vi "Configure Module.vi"(8 "error in (no error)":errorcluster, 10 "IOV ref in":refnum<k21>, 11 "Module Template in":refnum<class "9401.lvclass">) -> (0 "error out":errorcluster, 2 "IOV ref out":refnum<k21>, 3 "Module Template out":refnum<class "9401.lvclass">)   [LabVIEW 2017, in "Modules.lvlib" / "9401.lvclass"]
uses:
  9401.lvclass
  C:/Users/rzoeller/Documents/ni-official/niveristand-scan-engine-module-libraries/Source/SD Module/SD Module.lvclass
  9401.lvclass/9401.ctl
  SD Module/SD Module.lvclass
  <resource>/objmgr/cRIO.rc
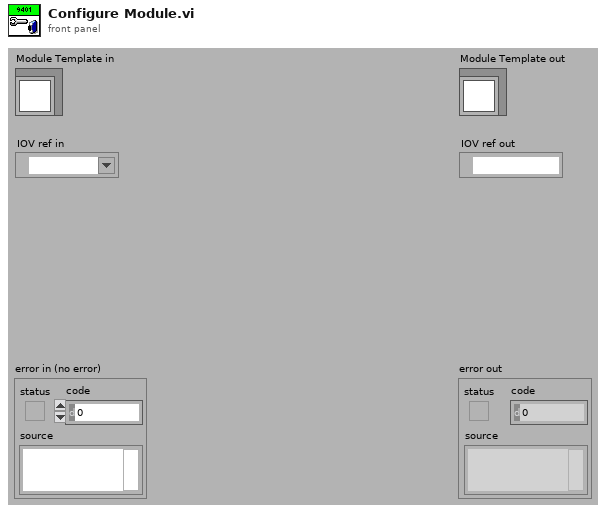
[diagram p1: front panel]
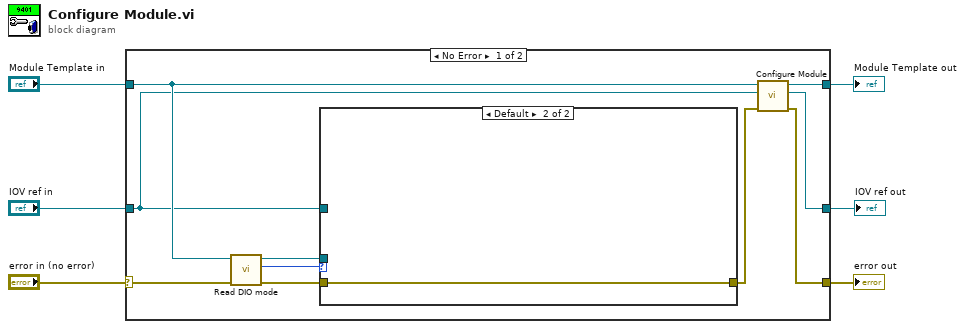
[diagram p0: block diagram]
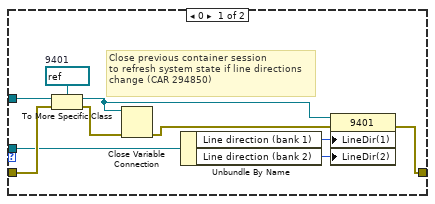
[diagram p2: hidden frame]
diagram:
  n1 = case shown="No Error" "error in (no error)" {
    selector: "error in (no error)" -> [w15 w30]
    tunnel: [w11 w30] -> w5
    tunnel: [w7 w29] -> w3
    tunnel: "Module Template in" -> [w10 w29]
    tunnel: "IOV ref in" -> [w9 w28]
    tunnel: [w8 w28] -> w1
    frame No Error {
      n2 = call "Read DIO mode.vi"("error in (no error)"=w15, "SD Module in"=w10) -> ("error out"=w13:errorcluster, "DIO mode"=w14:u32, "SD Module out"=w16:refnum<class "9401.lvclass">)  [unwired: 7 in]
      n3 = case shown="Default" w14 {
        tunnel: [w17 w27] -> w12
        tunnel: w9 -> [w25 _]
        tunnel: w16 -> [w18 _]
        tunnel: w13 -> [w19 w27]
        frame 0 {
          w26 = refnum<k21> refnum  # 9401
          # "Close previous container session\nto refresh system state if line directions\nchange (CAR 294850)"
          n4 = To More Specific Class(target class=w26, reference=w25, error in=w19) -> (specific class reference=w20:refnum<k21>, error out=w22:errorcluster)
          n5 = Close Variable Connection(8:w22, 11:w20) -> (0:w21:errorcluster)
          n6 = Unbundle By Name(w18) -> ("Line direction (bank 1)"=w24:u32, "Line direction (bank 2)"=w23:u32)
          n7 = property class="9401"(reference=w20, error in=w21, "LineDir(1)"=w24, "LineDir(2)"=w23) -> (error out=w17:errorcluster)  [unwired: 1 out]
        }
        frame Default {
        }
      }
      n8 = call-parent "Configure Module.vi"("error in (no error)"=w12, "IOV ref in"=w9, "Module Template in"=w10) -> ("error out"=w11:errorcluster, "IOV ref out"=w8:refnum<k21>, "Module Template out"=w7:refnum<class "9401.lvclass">)  [unwired: 6 in]
    }
    frame Error {
    }
  }
  "error out" <- w5
  "Module Template out" <- w3
  "IOV ref out" <- w1
